vi "Read Panel Info.vi"(10 "Runtime Implementation":T1) -> (1 "VI Refnum":refnum<vi>, 2 "Tab Name":string)   [LabVIEW 2015, in "E2E Tag Exchange editor node.lvclass"]
uses:
  E2E Tag Exchange editor node.lvclass
  module/configuration/Runtime Implementation.ctl
  UDP/UDP UI.vi
  module/configuration/E2E Tag Exchange configuration.lvclass
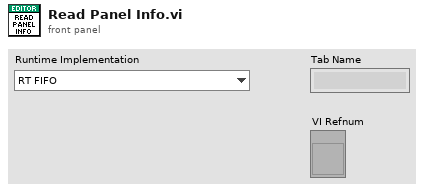
[diagram p1: front panel]
types:
  T1 = typedef "E2E Tag Exchange configuration.lvclass/Runtime Implementation.ctl" = enum16{"RT FIFO", "UDP"}
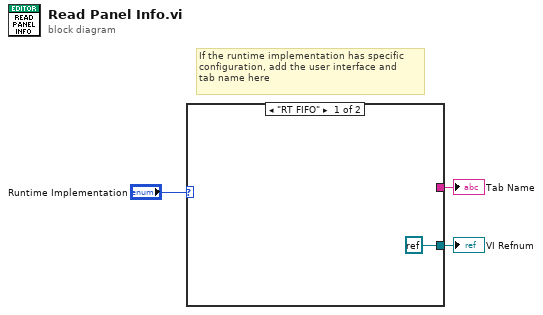
[diagram p0: block diagram]
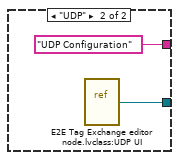
[diagram p2: hidden frame]
diagram:
  # "If the runtime implementation has specific\nconfiguration, add the user interface and\ntab name here"
  n1 = case shown="\"RT FIFO\"" "Runtime Implementation" {
    tunnel: [_ "UDP Configuration"] -> w2
    tunnel: [refnum<k0> refnum w5] -> w1
    frame "RT FIFO" {
    }
    frame "UDP" {
      n2 = vi-ref "E2E Tag Exchange editor node.lvclass:UDP UI.vi"() -> (w5:refnum<vi>)
    }
  }
  "Tab Name" <- w2
  "VI Refnum" <- w1
